vi "VideoFile.vi"(8 "error in (no error)":errorcluster, 10 "name":string, 11 "VideoFile in":refnum<class "VideoFile.lvclass">) -> (0 "error out":errorcluster, 3 "VideoFile out":refnum<class "VideoFile.lvclass">)   [LabVIEW 2017, in "VideoFile.lvclass"]
uses:
  VideoFile.lvclass
  VideoFile.lvclass/VideoFile.ctl
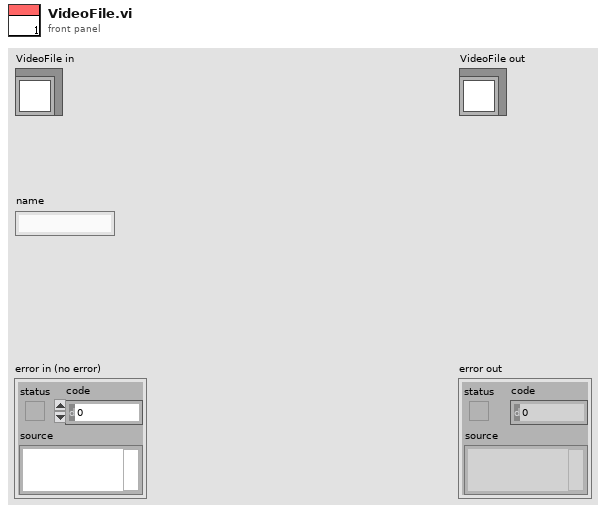
[diagram p1: front panel]
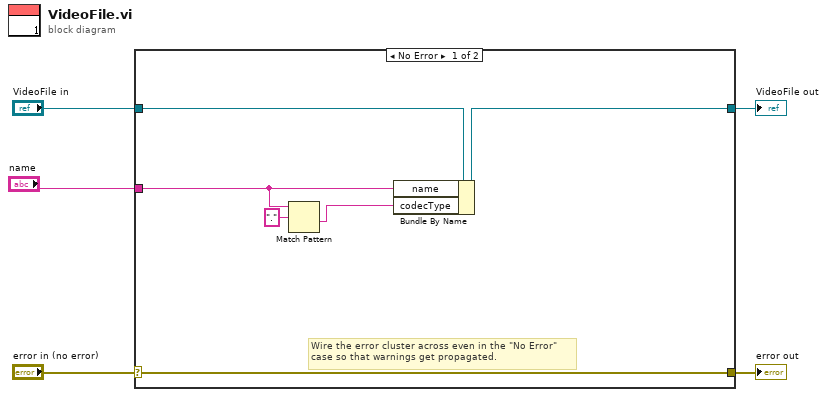
[diagram p0: block diagram]
diagram:
  n1 = case shown="No Error" "error in (no error)" {
    selector: "error in (no error)" -> [w10 w13]
    tunnel: [w10 w13] -> w4
    tunnel: [w9 w12] -> w2
    tunnel: "VideoFile in" -> [w11 w12]
    tunnel: "name" -> [w8 _]
    frame No Error {
      # "Wire the error cluster across even in the \"No Error\"\ncase so that warnings get propagated."
      n2 = Match Pattern(string=w8, regular expression=".") -> (after substring=w6:string)  [unwired: 1 in, 3 out]
      n3 = Bundle By Name(cluster=w11, "name"=w8, "codecType"=w6) -> (w9:refnum<class "VideoFile.lvclass">)
    }
    frame Error {
    }
  }
  "error out" <- w4
  "VideoFile out" <- w2
